vi "get reserving node by name.vi"(8 "error in (no error)":errorcluster, 10 "name":string, 11 "Item Ref in":T1 format="%.0x") -> (0 "error out":errorcluster, 1 "Dependent Node Ref":T1=18446744073709551615 format="%.0x", 3 "Item Ref out":T1 format="%.0x", 4 "Found":bool)   [LabVIEW 2016, in "FPGA RM System Definition API.lvlib"]
uses:
  System Definition/FPGA RM System Definition API.lvlib
  <vilib>/NI Veristand/Custom Device API/Custom Device Item Ref.ctl
  <vilib>/NI Veristand/Custom Device API/Get Item Property (Dependent Node Pointer).vi
  <vilib>/NI VeriStand/Custom Device API/Custom Device API.lvlib
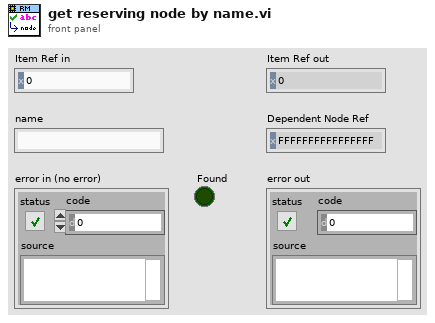
[diagram p1: front panel]
types:
  T1 = typedef "Custom Device API.lvlib/Custom Device Item Ref.ctl" = u64
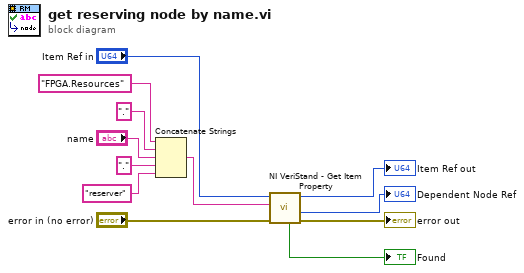
[diagram p0: block diagram]
diagram:
  n1 = Concatenate Strings("FPGA.Resources" ("string"), "." ("string"), "name", "." ("string"), "reserver" ("string")) -> (w12:string)
  n2 = call-poly <vilib>:"NI VeriStand - Get Item Property.vi"("error in (no error)"="error in (no error)", "Property Name"=w12, "Item Ref in"="Item Ref in") -> ("error out"=→"error out":errorcluster, "Dependent Node Ref"=→"Dependent Node Ref":T1, "Item Ref out"=→"Item Ref out":T1, "Found"=→"Found":bool)  [unwired: 5 in]
